vi "getArrayVisa.vi"() -> (1 "Size Array Visa":i32, 2 "Array Visa":refnum<visa-resource-name>[](array[refnum]))   [LabVIEW 2013]
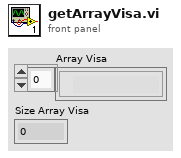
[diagram p1: front panel]
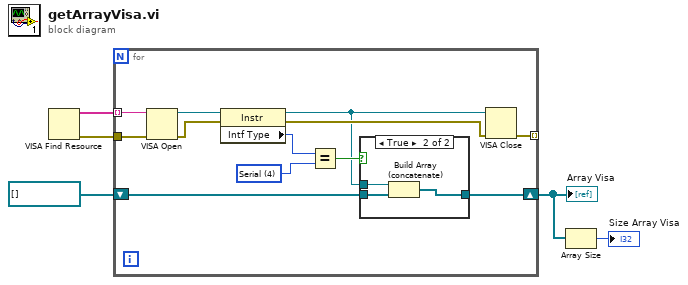
[diagram p0: block diagram]
diagram:
  n1 = VISA Find Resource() -> (0:w4:errorcluster, 3:w5:string[])  [unwired: 3 in, 1 out]
  n2 = for {
    tunnel: w5 -> [w17] mode=indexing
    tunnel: w4 -> [w16]
    tunnel: [w9] -> _ mode=indexing
    shift-right: [w6] -> w2
    shift-left: refnum<visa-resource-name>[] [] ("appended array") -> [w7]
    w12 = u16 4 items=["GPIB"=1, "VXI"=2, "GPIB-VXI"=3, "Serial"=4, "PXI"=5, "TCPIP"=6, "USB"=7, "FireWire"=9] ("Interface Information:Interface Type")
    n3 = VISA Open(error in (no error)=w16, VISA resource name=w17) -> (VISA resource name=w15:refnum<visa-resource-name>, error out=w14:errorcluster)  [unwired: 3 in]
    n4 = property class="Instr"(reference=w15, error in=w14) -> (reference out=w8:refnum<visa-resource-name>, error out=w10:errorcluster, "Intf Type"=w13:u16)
    n5 = Equal?(x=w13, y=w12) -> (x = y?=w11:bool)
    n6 = case shown="True" w11 {
      tunnel: w8 -> [_ w21]
      tunnel: w7 -> [w18 w20]
      tunnel: [w18 w19] -> w6
      frame False {
      }
      frame True {
        n7 = Build Array (concatenate)(w21, w20) -> (w19:refnum<visa-resource-name>[])
      }
    }
    n8 = VISA Close(VISA resource name=w8, error in (no error)=w10) -> (error out=w9:errorcluster)
  }
  "Array Visa" <- w2
  n9 = Array Size(array=w2) -> (size(s)=→"Size Array Visa":i32)
